vi "NATS CLI Install Windows.vi"() -> (0 "error out":errorcluster)   [LabVIEW 2020, in "NATS Infrastructure.lvlib"]
doc: "Starts NATS server on Windows machines."
uses:
  NATS Infrastructure.lvlib
panel:
  in  "Architecture":enum16{"amd64", "arm64", "386"}(ring)
  out "Return Code":i32
  out "Error":string
  out "Output":string
  in  "Install Directory":path=path "C:/nats"
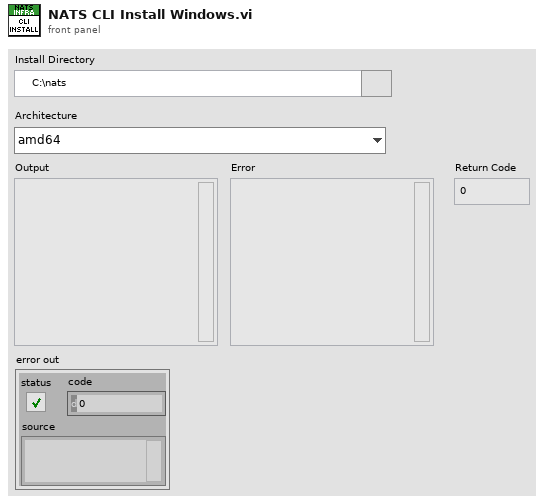
[diagram p1: front panel]
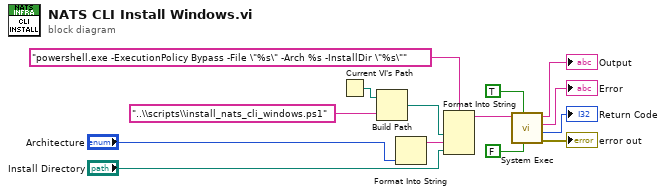
[diagram p0: block diagram]
diagram:
  n1 = Current VI's Path() -> (path=w9:path)
  n2 = Build Path(base path=w9, name or relative path="..\\scripts\\install_nats_cli_windows.ps1") -> (appended path=w8:path)
  n3 = Format Into String("Architecture") -> (resulting string=w1:string)  [unwired: 3 in, 1 out]
  n4 = Format Into String(format string="powershell.exe -ExecutionPolicy Bypass -File \"%s\" -Arch %s -InstallDir \"%s\"", w8, w1, "Install Directory") -> (resulting string=w7:string)  [unwired: 2 in, 1 out]
  n5 = call <vilib>:"System Exec.vi"("run minimized? (F)"=FALSE, "wait until completion? (T)"=TRUE, "command line"=w7) -> ("error out"=→"error out":errorcluster, "return code"=→"Return Code":i32, "standard error"=→"Error":string, "standard output"=→"Output":string)  [unwired: 5 in]
